vi "run.vi"(8 "error in (no error)":errorcluster, 11 "ScanHeadMH100729FPGA in":refnum<class "ScanHeadMH100729FPGA.lvclass">) -> (0 "error out":errorcluster, 3 "ScanHeadMH100729FPGA out":refnum<class "ScanHeadMH100729FPGA.lvclass">)   [LabVIEW 2010, in "ScanHeadMH100729FPGA.lvclass"]
uses:
  ScanHeadMH100729FPGA.lvclass
  intensity_adjustment_enum.ctl
  translation_mode_enum.ctl
  main/labview_source/controls/undock_button.ctl
  internal_trigger_enum.ctl
  ScanHeadMH100729FPGA.lvclass/ScanHeadMH100729FPGA.ctl
  GenericScanHead/GenericScanHead/GenericScanHead.lvclass
  Trajectory/GenericTrajectory/GenericTrajectory/GenericTrajectory.lvclass
  Trajectory/TrajectoryMG100122GenericFPGA/TrajectoryMG100122GenericFPGA/TrajectoryMG100122GenericFPGA.lvclass
  Objective/GenericObjective/GenericObjective/GenericObjective.lvclass
  <vilib>/Utility/inputDevices.llb/closeMouse.vi
  <vilib>/Utility/inputDevices.llb/closeKeyboard.vi
  common/classes/ErrorController/ErrorController/class_data.vi
  <vilib>/Utility/inputDevices.llb/mouseAcquire.vi
  <vilib>/Utility/inputDevices.llb/keyboardAcquire.vi
  common/classes/ErrorController/ErrorController/ErrorController.lvclass
panel:
  in  "button:undock":T1
  in  "Tab Control":enum32{"user", "debug", "about"}(tab)
  in  "modifyButton":bool
  in  "zoom":dbl(slide)=1.0 min=1.0 max=20.0 step=0.1 scale=1.0..20.0
  in  "offset tabs":enum32{"fine", "coarse"}(tab)
  in  "x offset":dbl[unit](slide) scale format="%#_3g"
  in  "z offset":dbl[unit](slide)
  in  "y offset":dbl[unit](slide) scale format="%#_3g"
  in  "zero offset":bool
  in  "zero angles":bool
  in  "laser intensity (%)":dbl(slide)=14.5 caption="intensity (%)" min=0.001 max=100.0 step=0.1 scale=0.0..100.0
  in  "intensity adjustment mode":T2=enum."look-up" caption="laser intensity\nadjustment"
  in  "scattering length":dbl[unit]=0.00019999999999999998 min=1e-10
  in  "z angle":dbl[unit](slide) min=0.0 max=6.283185307179586 step=0.01745329238474369
  in  "x angle":dbl[unit](slide) caption="X amplitude" min=0.0 max=3.141592653589793 step=0.01745329238474369
  in  "translation mode":T3
  in  "stop":bool
  out "evt lp error":errorcluster
  out "last trigger":T4
  out "state machine counter":i32
  # "translation"
  # "rotation & tilting"
  # "ScanHeadMH100729FPGA"
  # "Author: Marcel van 't Hoff, University of Zurich"
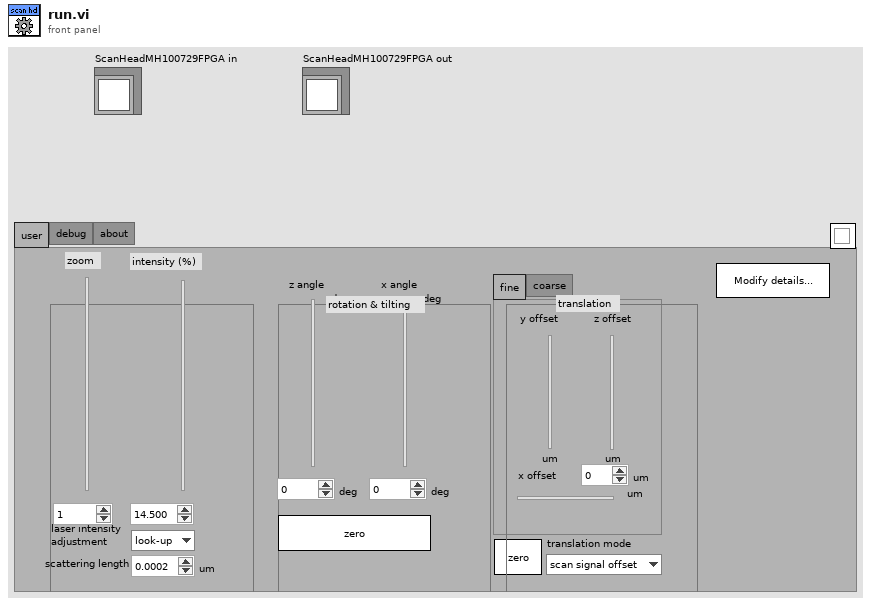
[diagram p1: front panel]
types:
  T1 = typedef "undock_button.ctl" = bool
  T2 = typedef "ScanHeadMH100729FPGA.lvclass/intensity_adjustment_enum.ctl" = enum16{"manual", "look-up", "exponential"}
  T3 = typedef "ScanHeadMH100729FPGA.lvclass/translation_mode_enum.ctl" = enum16{"scan signal offset", "stage"}
  T4 = typedef "ScanHeadMH100729FPGA.lvclass/internal_trigger_enum.ctl" = enum16{"NULL", "initialise", "terminate", "start scanning", "stop scanning", "update", "fetch trajectory", "update bounding box"}
  T5 = cluster{"Horizontal":i32, "Vertical":i32, "Scrolling":i32}
  T6 = enum16{"0", "1", "2", "3", "4", "5", "6", "7", "8", "9", "A", "B", "C", "D", "E", "F", "G", "H", "I", "J", "K", "L", "M", "N", "O", "P", "Q", "R", "S", "T", "U", "V", "W", "X", "Y", "Z", "F1", "F2", "F3", "F4", "F5", "F6", "F7", "F8", "F9", "F10", "F11", "F12", "F13", "F14", "F15", "ADD", "BACK", "BACKSLASH", "CAPITAL", "COMMA", "DECIMAL", "DELETE", "DIVIDE", "DOWN", "END", "EQUALS", "ESCAPE", "GRAVE (`)", "HOME", "INSERT", "LBRACKET", "LCONTROL", "LEFT", "L ALT", "LSHIFT", "LWIN", "MINUS", "MULTIPLY", "NEXT", "NUMLOCK", "NUMPAD_0", "NUMPAD_1", "NUMPAD_2", "NUMPAD_3", "NUMPAD_4", "NUMPAD_5", "NUMPAD_6", "NUMPAD_7", "NUMPAD_8", "NUMPAD_9", "PAUSE", "PERIOD", "PRIOR (PG UP)", "RBRACKET", "RCONTROL", "RETURN", "RIGHT", "R ALT", "RSHIFT", "RWIN", "SCROLL", "SEMICOLON", "SLASH", "SPACE", "SUBTRACT", "TAB", "UP", "ENTER (num pad)", "' (quote)"}[]
  T7 = typedef "top-level_component_type_enum.ctl" = enum16{"undefined", "ImagingMode", "ScanHead", "DAQ", "ImageAssembler", "Display", "DataCollection", "Analyser", "Stimulator", "ExperimentController", "Instrument", "Stage"}
  T8 = typedef "main_trigger_enum.ctl" = enum16{"NULL", "initialise", "terminate", "start", "stop", "change objective", "change experimentController", "change imagingMode", "save notebook", "started saving", "finished saving", "expCtr ready", "expCtr missing", "imgMd ready", "imgMd missing", "scanHd ready", "scanHd missing", "DAQ ready", "DAQ missing", "imgAsm ready", "imgAsm missing", "dataColl ready", "dataColl missing", "display ready", "display missing", "analysr ready", "analysr missing", "instrmnt ready", "instrmnt missing", "stimltr ready", "stimltr missing", "stage ready", "stage missing"}
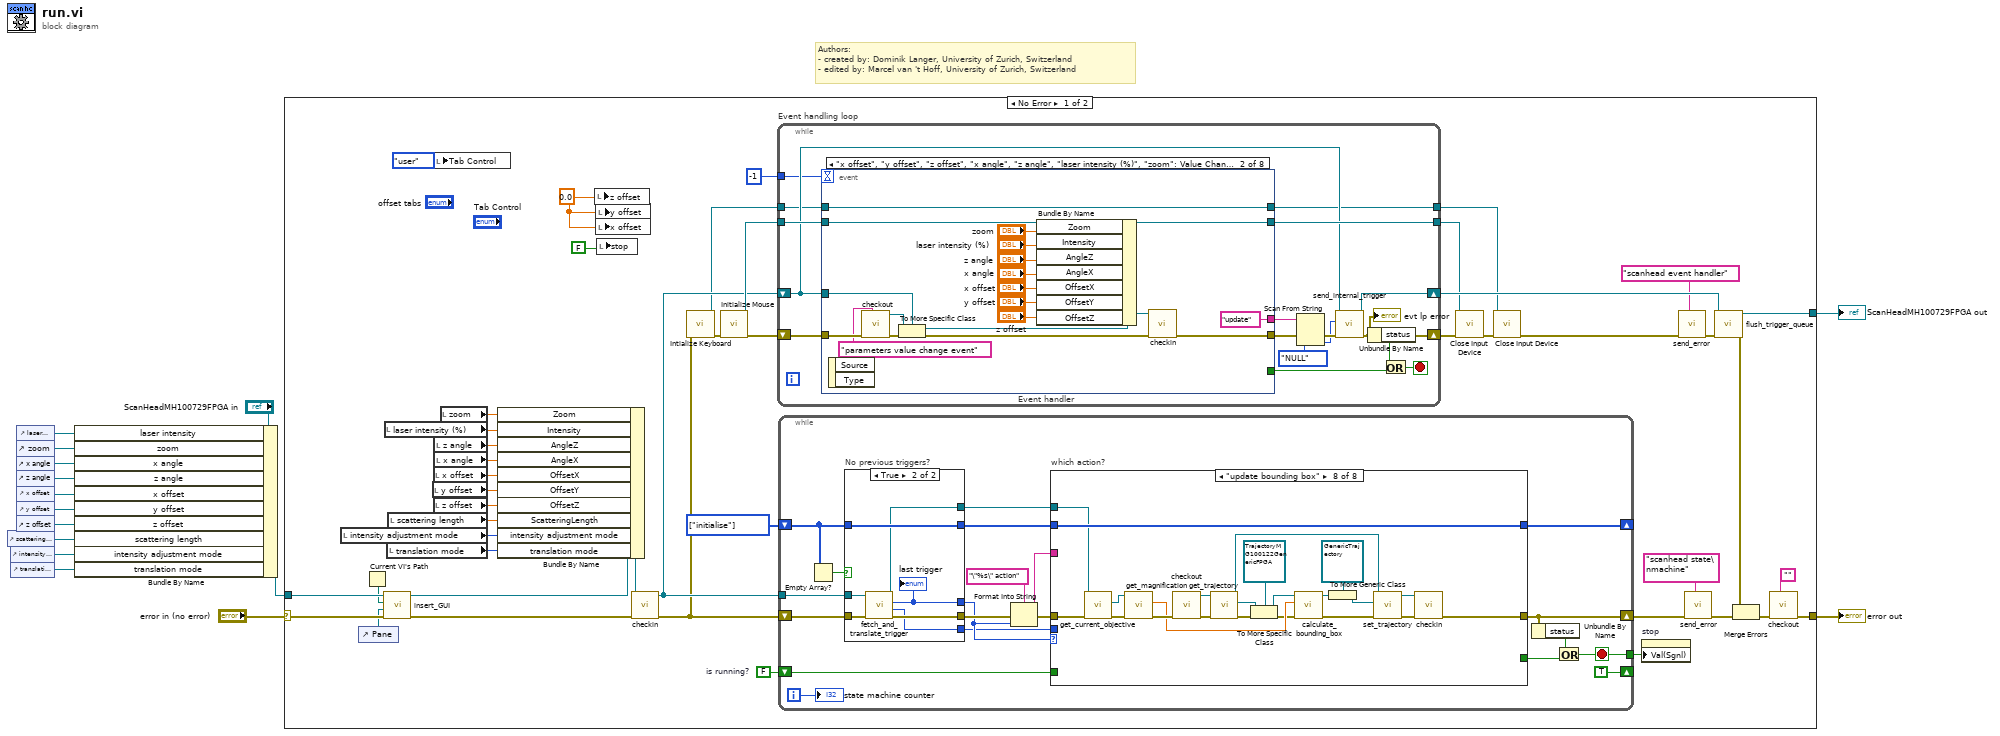
[diagram p0: block diagram]
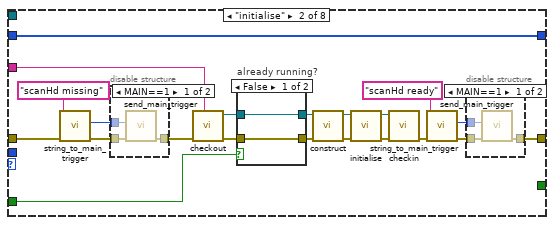
[diagram p3: hidden frame]
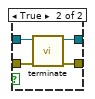
[diagram p5: hidden frame]
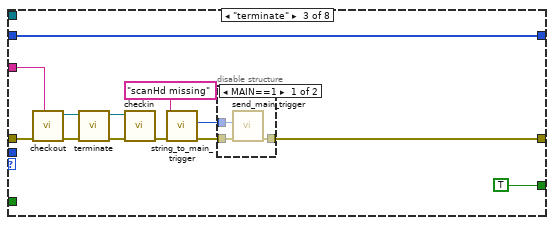
[diagram p7: hidden frame]
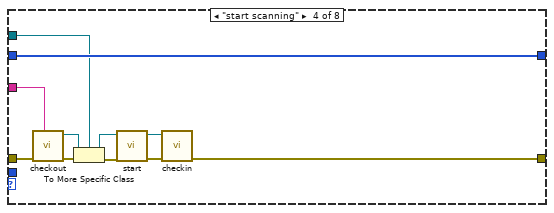
[diagram p9: hidden frame]
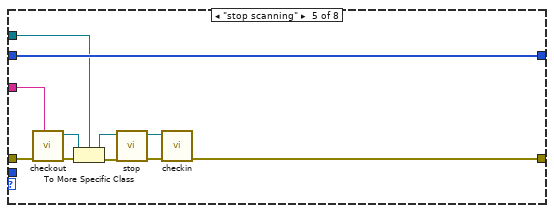
[diagram p10: hidden frame]
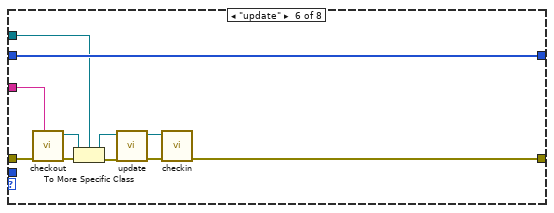
[diagram p11: hidden frame]
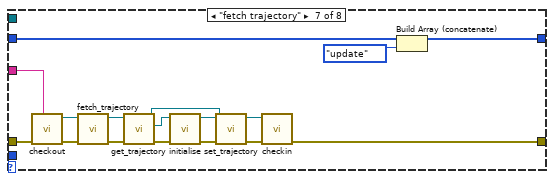
[diagram p12: hidden frame]
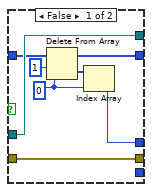
[diagram p13: hidden frame]
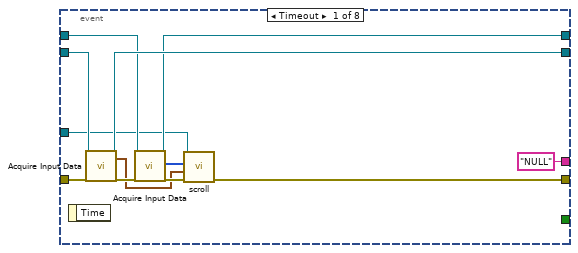
[diagram p14: hidden frame]
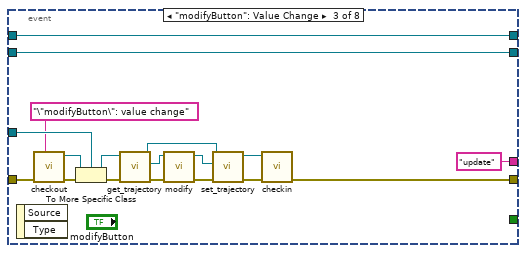
[diagram p15: hidden frame]
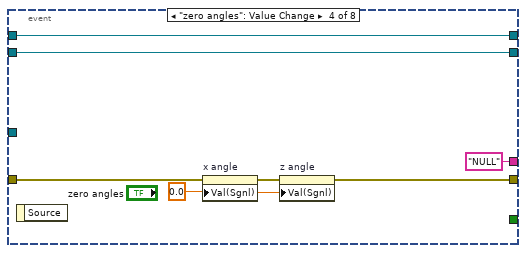
[diagram p16: hidden frame]
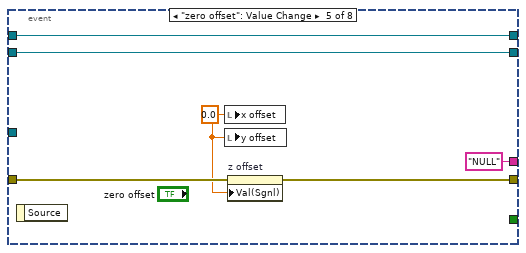
[diagram p17: hidden frame]
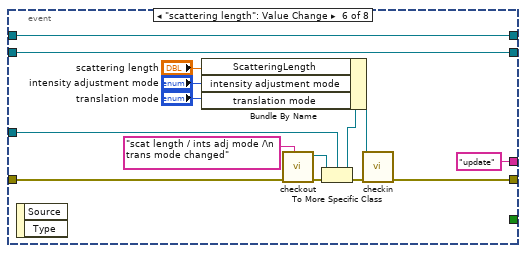
[diagram p18: hidden frame]
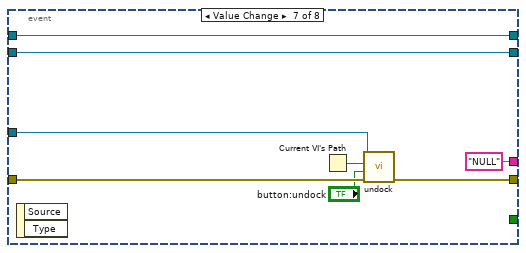
[diagram p19: hidden frame]
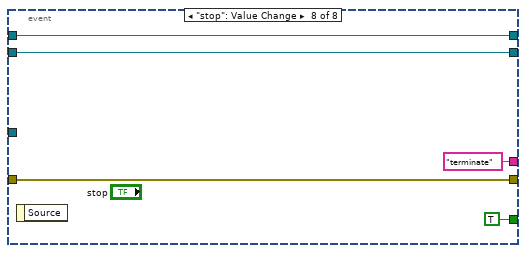
[diagram p20: hidden frame]
diagram:
  # "Authors: \n- created by: Dominik Langer, University of Zurich, Switzerland\n- edited by: Marcel van 't Hoff, University of Zurich, Switzerland"
  n1 = control-ref of="scattering length"() -> (w10:refnum<vi>)
  n2 = control-ref of="intensity adjustment mode"() -> (w9:refnum<vi>)
  n3 = control-ref of="translation mode"() -> (w3:refnum<vi>)
  n4 = control-ref of="laser intensity (%)"() -> (w8:refnum<vi>)
  n5 = control-ref of="zoom"() -> (w13:refnum<vi>)
  n6 = control-ref of="x angle"() -> (w11:refnum<vi>)
  n7 = control-ref of="z angle"() -> (w12:refnum<vi>)
  n8 = control-ref of="x offset"() -> (w5:refnum<vi>)
  n9 = control-ref of="y offset"() -> (w6:refnum<vi>)
  n10 = control-ref of="z offset"() -> (w7:refnum<vi>)
  n11 = Bundle By Name(cluster="ScanHeadMH100729FPGA in", "laser intensity"=w8, "zoom"=w13, "x angle"=w11, "z angle"=w12, "x offset"=w5, "y offset"=w6, "z offset"=w7, "scattering length"=w10, "intensity adjustment mode"=w9, "translation mode"=w3) -> (w14:refnum<class "ScanHeadMH100729FPGA.lvclass">)
  n12 = case shown="No Error" "error in (no error)" {
    selector: "error in (no error)" -> [w44 w331]
    tunnel: [w60 w331] -> w4
    tunnel: [w37 w330] -> w1
    tunnel: w14 -> [w43 w330]
    frame No Error {
      w29 = FALSE  # is running?
      w30 = T4[] [enum."initialise"] items=["NULL", "initialise", "terminate", "start scanning", "stop scanning", "update", "fetch trajectory", "update bounding box"]
      w56 = dbl[unit] 0.0 ("z offset")
      n13 = local read "intensity adjustment mode"() -> (w51:T2)
      n14 = control-ref of="Pane"() -> (w39:refnum<vi>)
      n15 = Current VI's Path() -> (path=w42:path)
      n16 = call-dynamic "insert_GUI.vi"("error in (no error)"=w44, "Pane"=w39, "VI path"=w42, "GenericComponent in"=w43) -> ("error out"=w16:errorcluster, "GenericComponent out"=w35:refnum<class "ScanHeadMH100729FPGA.lvclass">)  [unwired: 6 in]
      n17 = local read "laser intensity (%)"() -> (w53:dbl)
      n18 = local read "translation mode"() -> (w41:T3)
      n19 = local read "scattering length"() -> (w50:dbl[unit])
      n20 = local read "y offset"() -> (w46:dbl[unit])
      n21 = local read "x offset"() -> (w47:dbl[unit])
      n22 = local read "z offset"() -> (w45:dbl[unit])
      n23 = local write "Tab Control"(enum32{"user", "debug", "about"}."user" ("Tab Control")) -> ()
      n24 = local read "z angle"() -> (w49:dbl[unit])
      n25 = local read "x angle"() -> (w48:dbl[unit])
      n26 = local read "zoom"() -> (w54:dbl)
      n27 = Bundle By Name(cluster=w35, "Zoom"=w54, "Intensity"=w53, "AngleZ"=w49, "AngleX"=w48, "OffsetX"=w47, "OffsetY"=w46, "OffsetZ"=w45, "ScatteringLength"=w50, "intensity adjustment mode"=w51, "translation mode"=w41) -> (w52:refnum<class "ScanHeadMH100729FPGA.lvclass">)
      n28 = local write "z offset"(w56) -> ()
      n29 = local write "y offset"(w56) -> ()
      n30 = local write "x offset"(w56) -> ()
      n31 = local write "stop"(FALSE) -> ()
      n32 = call-dynamic "checkin.vi"("error in (no error)"=w16, "GenericScanHead in"=w52) -> ("error out"=w28:errorcluster, "GenericScanHead out"=w32:refnum<class "ScanHeadMH100729FPGA.lvclass">)  [unwired: 8 in]
      n33 = call <vilib>:"Intialize Keyboard.vi"("error in (no error)"=w28) -> ("error out"=w27:errorcluster, "device ID"=w26:refnum<k1>)  [unwired: 9 in]
      n34 = call <vilib>:"Initialize Mouse.vi"("error in (no error)"=w27) -> ("error out"=w55:errorcluster, "device ID"=w59:refnum<k1>)  [unwired: 9 in]
      n35 = while "Event handling loop" {
        shift-right: [w234] -> w21
        shift-left: w55 -> [w239]
        tunnel: w59 -> [w238]
        tunnel: [w237] -> w24
        shift-right: [w236] -> w36
        shift-left: w32 -> [w235]
        tunnel: w26 -> [w230]
        tunnel: [w229] -> w23
        tunnel: -1 -> [w228]
        stop <- w231 stop-if-true
        n36 = event "Event handler" shown="[1] \"x offset\", \"y offset\", \"z offset\", \"x angle\", \"z angle\", \"laser intensity (%)\", \"zoom\": Value Change" {
          selector: _ -> [_ _ _ _ _ _ _ _]
          dyn-events: _ -> [_ _ _ _ _ _ _ _]
          timeout: w228 -> [_ _ _ _ _ _ _ _]
          tunnel: w239 -> [w249 w268 w287 w295 w301 w306 w322 w329]
          tunnel: [w243 w258 w280 w293 w300 w305 w321 w329] -> w225
          tunnel: [_ _ _ _ _ _ _ TRUE] -> w232
          tunnel: w235 -> [w244 w267 w284 _ _ w312 w323 _]
          tunnel: w238 -> [w251 w270 w288 w291 w298 w316 w324 w327]
          tunnel: [w250 w270 w288 w291 w298 w316 w324 w327] -> w237
          tunnel: w230 -> [w247 w253 w272 w290 w297 w303 w318 w326]
          tunnel: [w246 w253 w272 w290 w297 w303 w318 w326] -> w229
          tunnel: ["NULL" "update" "update" "NULL" "NULL" "update" "NULL" "terminate"] -> w223
          event Timeout {
            n37 = event-data() -> ()  [unwired: 2 out]
            n38 = call-poly <vilib>:"Acquire Input Data.vi"("device ID"=w251, "error in (no error)"=w249) -> ("device ID"=w250:refnum<k1>, "axis info"=w241:T5, "error out"=w248:errorcluster)  [unwired: 14 in, 1 out]
            n39 = call-poly <vilib>:"Acquire Input Data.vi"("device ID"=w247, "error in (no error)"=w248) -> ("device ID"=w246:refnum<k1>, "keys pressed"=w242:T6, "error out"=w245:errorcluster)  [unwired: 15 in]
            n40 = call-dynamic "scroll.vi"("error in (no error)"=w245, "axis info"=w241, "keys pressed"=w242, "ScanHeadMH100729FPGA in"=w244) -> ("error out"=w243:errorcluster)  [unwired: 6 in, 1 out]
          }
          event "x offset", "y offset", "z offset", "x angle", "z angle", "laser intensity (%)", "zoom": Value Change {
            n41 = event-data() -> ()  [unwired: 3 out]
            n42 = call "checkout.vi"("locked by?"="parameters value change event", "error in (no error)"=w268) -> ("error out"=w269:errorcluster, "GenericScanHead out"=w266:refnum<class "GenericScanHead.lvclass">)  [unwired: 8 in]
            n43 = To More Specific Class(target class=w267, reference=w266, error in=w269) -> (specific class reference=w264:refnum<class "ScanHeadMH100729FPGA.lvclass">, error out=w259:errorcluster)
            n44 = Bundle By Name(cluster=w264, "Zoom"="zoom", "Intensity"="laser intensity (%)", "AngleZ"="z angle", "AngleX"="x angle", "OffsetX"="x offset", "OffsetY"="y offset", "OffsetZ"="z offset") -> (w257:refnum<class "ScanHeadMH100729FPGA.lvclass">)
            n45 = call-dynamic "checkin.vi"("error in (no error)"=w259, "GenericScanHead in"=w257) -> ("error out"=w258:errorcluster)  [unwired: 8 in, 1 out]
          }
          event "modifyButton": Value Change {
            n46 = event-data() -> ()  [unwired: 3 out]
            n47 = call "checkout.vi"("locked by?"="\"modifyButton\": value change", "error in (no error)"=w287) -> ("error out"=w286:errorcluster, "GenericScanHead out"=w285:refnum<class "GenericScanHead.lvclass">)  [unwired: 8 in]
            n48 = To More Specific Class(target class=w284, reference=w285, error in=w286) -> (specific class reference=w283:refnum<class "ScanHeadMH100729FPGA.lvclass">, error out=w282:errorcluster)
            n49 = call-dynamic "get_trajectory.vi"("error in (no error)"=w282, "GenericScanHead.lvclass in"=w283) -> ("error out"=w276:errorcluster, "trajectory"=w274:refnum<class "GenericTrajectory.lvclass">, "GenericScanHead.lvclass out"=w278:refnum<class "ScanHeadMH100729FPGA.lvclass">)  [unwired: 7 in]
            n50 = call-dynamic "modify.vi"("error in (no error)"=w276, "GenericTrajectory in"=w274) -> ("error out"=w275:errorcluster, "GenericTrajectory out"=w273:refnum<class "GenericTrajectory.lvclass">)  [unwired: 8 in]
            n51 = call-dynamic "set_trajectory.vi"("error in (no error)"=w275, "trajectory"=w273, "GenericScanHead.lvclass in"=w278) -> ("error out"=w281:errorcluster, "GenericScanHead.lvclass out"=w279:refnum<class "ScanHeadMH100729FPGA.lvclass">)  [unwired: 7 in]
            n52 = call-dynamic "checkin.vi"("error in (no error)"=w281, "GenericScanHead in"=w279) -> ("error out"=w280:errorcluster)  [unwired: 8 in, 1 out]
          }
          event "zero angles": Value Change {
            w292 = dbl[unit] 0.0 ("Value (Signaling)")
            n53 = event-data() -> ()  [unwired: 2 out]
            n54 = property on="x angle" class="Slide (strict)"(error in=w295, "Val(Sgnl)"=w292) -> (error out=w294:errorcluster)  [unwired: 1 in, 1 out]
            n55 = property on="z angle" class="Slide (strict)"(error in=w294, "Val(Sgnl)"=w292) -> (error out=w293:errorcluster)  [unwired: 1 in, 1 out]
          }
          event "zero offset": Value Change {
            w299 = dbl[unit] 0.0 ("x offset")
            n56 = event-data() -> ()  [unwired: 2 out]
            n57 = local write "x offset"(w299) -> ()
            n58 = local write "y offset"(w299) -> ()
            n59 = property on="z offset" class="Slide (strict)"(error in=w301, "Val(Sgnl)"=w299) -> (error out=w300:errorcluster)  [unwired: 1 in, 1 out]
          }
          event "scattering length": Value Change {
            n60 = event-data() -> ()  [unwired: 3 out]
            n61 = call "checkout.vi"("locked by?"="scat length / ints adj mode /\n trans mode changed", "error in (no error)"=w306) -> ("error out"=w309:errorcluster, "GenericScanHead out"=w311:refnum<class "GenericScanHead.lvclass">)  [unwired: 8 out]
            n62 = To More Specific Class(target class=w312, reference=w311, error in=w309) -> (specific class reference=w310:refnum<class "ScanHeadMH100729FPGA.lvclass">, error out=w308:errorcluster)
            n63 = Bundle By Name(cluster=w310, "ScatteringLength"="scattering length", "intensity adjustment mode"="intensity adjustment mode", "translation mode"="translation mode") -> (w307:refnum<class "ScanHeadMH100729FPGA.lvclass">)
            n64 = call-dynamic "checkin.vi"("error in (no error)"=w308, "GenericScanHead in"=w307) -> ("error out"=w305:errorcluster)  [unwired: 8 in, 1 out]
          }
          event Value Change {
            n65 = event-data() -> ()  [unwired: 3 out]
            n66 = Current VI's Path() -> (path=w319:path)
            n67 = call-dynamic "undock.vi"("error in (no error)"=w322, "undock?"="button:undock", "VI path"=w319, "component in"=w323) -> ("error out"=w321:errorcluster)  [unwired: 6 in, 1 out]
          }
          event "stop": Value Change {
            n68 = event-data() -> ()  [unwired: 2 out]
          }
        }
        n69 = Scan From String(input string=w223, error in=w225, default 1=internal_trigger_enum."NULL" ("trigger")) -> (error out=w226:errorcluster, output 1=w224:T4)  [unwired: 2 in, 2 out]
        n70 = call-dynamic "send_internal_trigger.vi"("error in (no error)"=w226, "trigger"=w224, "ScanHeadMH100729FPGA in"=w235) -> ("error out"=w234:errorcluster, "ScanHeadMH100729FPGA out"=w236:refnum<class "ScanHeadMH100729FPGA.lvclass">)  [unwired: 7 in]
        "evt lp error" <- w234
        n71 = Unbundle By Name(w234) -> ("status"=w233:bool)
        n72 = Or(x=w233, y=w232) -> (x .or. y?=w231:bool)
      }
      n73 = while {
        shift-right: [w66] -> w31
        shift-left: w28 -> [w81]
        shift-right: [w72] -> _
        shift-left: w30 -> [w78]
        shift-right: [TRUE ("is running?")] -> _
        shift-left: w29 -> [w69]
        tunnel: w32 -> [w80]
        tunnel: [w64] -> w18
        i -> [w62]
        stop <- w64 stop-if-true
        n74 = Empty Array?(array=w78) -> (empty?=w79:bool)
        n75 = case "No previous triggers?" shown="True" w79 {
          tunnel: w80 -> [w215 w220]
          tunnel: w81 -> [w213 w221]
          tunnel: [w215 w219] -> w73
          tunnel: [w211 w216] -> w75
          tunnel: [_ w217] -> w67
          tunnel: [w213 w218] -> w76
          tunnel: w78 -> [w214 w222]
          tunnel: [w210 w222] -> w71
          frame False {
            w208 = 0 ("index")
            n76 = Delete From Array(array=w214, length=1, index=w208) -> (deleted portion=w212:T4[], array with subset deleted=w210:T4[])
            n77 = Index Array(array=w212, index=w208) -> (element=w211:T4)
          }
          frame True {
            n78 = call-dynamic "fetch_and_translate_trigger.vi"("error in (no error)"=w221, "ScanHeadMH100729FPGA in"=w220) -> ("error out"=w218:errorcluster, "sender TLC type"=w217:T7, "internal trigger"=w216:T4, "ScanHeadMH100729FPGA out"=w219:refnum<class "ScanHeadMH100729FPGA.lvclass">)  [unwired: 6 in]
            "last trigger" <- w216
          }
        }
        n79 = Format Into String(format string="\"%s\" action", error in=w76, w75) -> (resulting string=w70:string, error out=w74:errorcluster)  [unwired: 1 in]
        n80 = case "which action?" shown="\"update bounding box\"" w75 {
          tunnel: [w82 w98 w119 w141 w152 w158 w179 w199] -> w66
          tunnel: w74 -> [w82 w85 w128 w142 w153 w164 w180 w205]
          tunnel: w73 -> [_ _ _ w138 w149 w161 _ w206]
          tunnel: [w83 w104 w131 w146 w157 w168 w170 w207] -> w72
          tunnel: w71 -> [w83 w104 w131 w146 w157 w168 w171 w207]
          tunnel: w70 -> [_ w99 w127 w140 w151 w163 w172 _]
          tunnel: w69 -> [_ w94 _ _ _ _ _ _]
          tunnel: w67 -> [_ _ _ _ _ _ _ _]
          tunnel: [_ _ TRUE _ _ _ _ _] -> w63
          frame "NULL", Default {
          }
          frame "initialise" {
            n81 = call "string_to_main_trigger.vi"("error in (no error)"=w85, "trigger string"="scanHd missing") -> ("error out"=w87:errorcluster, "main trigger"=w88:T8)  [unwired: 8 in]
            n82 = disable-structure shown="MAIN==1" {
              disable-tunnel: w87 -> [w107 w108]
              disable-tunnel: [w106 w108] -> w84
              disable-tunnel: w88 -> [w105 _]
              frame condition #0 {
                n83 = call "send_main_trigger.vi"("error in (no error)"=w107, "trigger"=w105) -> ("error out"=w106:errorcluster)  [unwired: 9 in]
              }
              frame condition #1 (active) {
              }
            }
            n84 = call "checkout.vi"("locked by?"=w99, "error in (no error)"=w84) -> ("error out"=w96:errorcluster, "GenericScanHead out"=w95:refnum<class "GenericScanHead.lvclass">)  [unwired: 8 in]
            n85 = case "already running?" shown="False" w94 {
              tunnel: [w110 w112] -> w97
              tunnel: w96 -> [w110 w111]
              tunnel: w95 -> [w109 w114]
              tunnel: [w109 w113] -> w93
              frame False {
              }
              frame True {
                n86 = call-dynamic "terminate.vi"("error in (no error)"=w111, "GenericPlugin in"=w114) -> ("error out"=w112:errorcluster, "GenericPlugin out"=w113:refnum<class "GenericScanHead.lvclass">)  [unwired: 8 out]
              }
            }
            n87 = call-dynamic "construct.vi"("error in (no error)"=w97, "GenericPlugin in"=w93) -> ("error out"=w101:errorcluster, "GenericPlugin out"=w102:refnum<class "GenericScanHead.lvclass">)  [unwired: 8 in]
            n88 = call-dynamic "initialise.vi"("error in (no error)"=w101, "GenericPlugin in"=w102) -> ("error out"=w100:errorcluster, "GenericPlugin out"=w103:refnum<class "GenericScanHead.lvclass">)  [unwired: 8 in]
            n89 = call-dynamic "checkin.vi"("error in (no error)"=w100, "GenericScanHead in"=w103) -> ("error out"=w92:errorcluster)  [unwired: 8 in, 1 out]
            n90 = call "string_to_main_trigger.vi"("error in (no error)"=w92, "trigger string"="scanHd ready") -> ("error out"=w91:errorcluster, "main trigger"=w89:T8)  [unwired: 8 in]
            n91 = disable-structure shown="MAIN==1" {
              disable-tunnel: w91 -> [w117 w118]
              disable-tunnel: [w116 w118] -> w98
              disable-tunnel: w89 -> [w115 _]
              frame condition #0 {
                n92 = call "send_main_trigger.vi"("error in (no error)"=w117, "trigger"=w115) -> ("error out"=w116:errorcluster)  [unwired: 9 in]
              }
              frame condition #1 (active) {
              }
            }
          }
          frame "terminate" {
            n93 = call "checkout.vi"("locked by?"=w127, "error in (no error)"=w128) -> ("error out"=w130:errorcluster, "GenericScanHead out"=w125:refnum<class "GenericScanHead.lvclass">)  [unwired: 8 in]
            n94 = call-dynamic "terminate.vi"("error in (no error)"=w130, "GenericPlugin in"=w125) -> ("error out"=w129:errorcluster, "GenericPlugin out"=w126:refnum<class "GenericScanHead.lvclass">)  [unwired: 8 in]
            n95 = call-dynamic "checkin.vi"("error in (no error)"=w129, "GenericScanHead in"=w126) -> ("error out"=w120:errorcluster)  [unwired: 8 in, 1 out]
            n96 = call "string_to_main_trigger.vi"("error in (no error)"=w120, "trigger string"="scanHd missing") -> ("error out"=w122:errorcluster, "main trigger"=w123:T8)  [unwired: 8 in]
            n97 = disable-structure shown="MAIN==1" {
              disable-tunnel: w122 -> [w134 w135]
              disable-tunnel: [w133 w135] -> w119
              disable-tunnel: w123 -> [w132 _]
              frame condition #0 {
                n98 = call "send_main_trigger.vi"("error in (no error)"=w134, "trigger"=w132) -> ("error out"=w133:errorcluster)  [unwired: 9 in]
              }
              frame condition #1 (active) {
              }
            }
          }
          frame "start scanning" {
            n99 = call "checkout.vi"("locked by?"=w140, "error in (no error)"=w142) -> ("error out"=w145:errorcluster, "GenericScanHead out"=w139:refnum<class "GenericScanHead.lvclass">)  [unwired: 8 in]
            n100 = To More Specific Class(target class=w138, reference=w139, error in=w145) -> (specific class reference=w137:refnum<class "ScanHeadMH100729FPGA.lvclass">, error out=w144:errorcluster)
            n101 = call-dynamic "start.vi"("error in (no error)"=w144, "ScanHeadMH100729FPGA in"=w137) -> ("error out"=w143:errorcluster, "ScanHeadMH100729FPGA out"=w136:refnum<class "ScanHeadMH100729FPGA.lvclass">)  [unwired: 8 in]
            n102 = call-dynamic "checkin.vi"("error in (no error)"=w143, "GenericScanHead in"=w136) -> ("error out"=w141:errorcluster)  [unwired: 8 in, 1 out]
          }
          frame "stop scanning" {
            n103 = call "checkout.vi"("locked by?"=w151, "error in (no error)"=w153) -> ("error out"=w156:errorcluster, "GenericScanHead out"=w150:refnum<class "GenericScanHead.lvclass">)  [unwired: 8 in]
            n104 = To More Specific Class(target class=w149, reference=w150, error in=w156) -> (specific class reference=w148:refnum<class "ScanHeadMH100729FPGA.lvclass">, error out=w155:errorcluster)
            n105 = call-dynamic "stop.vi"("error in (no error)"=w155, "ScanHeadMH100729FPGA in"=w148) -> ("error out"=w154:errorcluster, "ScanHeadMH100729FPGA out"=w147:refnum<class "ScanHeadMH100729FPGA.lvclass">)  [unwired: 8 in]
            n106 = call-dynamic "checkin.vi"("error in (no error)"=w154, "GenericScanHead in"=w147) -> ("error out"=w152:errorcluster)  [unwired: 8 in, 1 out]
          }
          frame "update" {
            n107 = call "checkout.vi"("locked by?"=w163, "error in (no error)"=w164) -> ("error out"=w167:errorcluster, "GenericScanHead out"=w162:refnum<class "GenericScanHead.lvclass">)  [unwired: 8 in]
            n108 = To More Specific Class(target class=w161, reference=w162, error in=w167) -> (specific class reference=w160:refnum<class "ScanHeadMH100729FPGA.lvclass">, error out=w166:errorcluster)
            n109 = call-dynamic "update.vi"("error in (no error)"=w166, "ScanHeadMH100729FPGA in"=w160) -> ("error out"=w165:errorcluster, "ScanHeadMH100729FPGA out"=w159:refnum<class "ScanHeadMH100729FPGA.lvclass">)  [unwired: 8 in]
            n110 = call-dynamic "checkin.vi"("error in (no error)"=w165, "GenericScanHead in"=w159) -> ("error out"=w158:errorcluster)  [unwired: 8 in, 1 out]
          }
          frame "fetch trajectory" {
            n111 = call "checkout.vi"("locked by?"=w172, "error in (no error)"=w180) -> ("error out"=w181:errorcluster, "GenericScanHead out"=w178:refnum<class "GenericScanHead.lvclass">)  [unwired: 8 in]
            n112 = call-dynamic "fetch_trajectory.vi"("error in (no error)"=w181, "GenericScanHead in"=w178) -> ("error out"=w182:errorcluster, "GenericScanHead out"=w177:refnum<class "GenericScanHead.lvclass">)  [unwired: 8 in]
            n113 = call-dynamic "get_trajectory.vi"("error in (no error)"=w182, "GenericScanHead.lvclass in"=w177) -> ("error out"=w183:errorcluster, "trajectory"=w175:refnum<class "GenericTrajectory.lvclass">, "GenericScanHead.lvclass out"=w176:refnum<class "GenericScanHead.lvclass">)  [unwired: 7 in]
            n114 = call-dynamic "initialise.vi"("error in (no error)"=w183, "GenericPlugin in"=w175) -> ("error out"=w184:errorcluster, "GenericPlugin out"=w174:refnum<class "GenericTrajectory.lvclass">)  [unwired: 8 in]
            n115 = call-dynamic "set_trajectory.vi"("error in (no error)"=w184, "trajectory"=w174, "GenericScanHead.lvclass in"=w176) -> ("error out"=w185:errorcluster, "GenericScanHead.lvclass out"=w173:refnum<class "GenericScanHead.lvclass">)  [unwired: 7 in]
            n116 = call-dynamic "checkin.vi"("error in (no error)"=w185, "GenericScanHead in"=w173) -> ("error out"=w179:errorcluster)  [unwired: 8 in, 1 out]
            n117 = Build Array (concatenate)(w171, internal_trigger_enum."update" ("last trigger")) -> (w170:T4[])
          }
          frame "update bounding box" {
            n118 = call-dynamic "get_current_objective.vi"("error in (no error)"=w205, "GenericPlugin in"=w206) -> ("error out"=w203:errorcluster, "current objective"=w204:refnum<class "GenericObjective.lvclass">)  [unwired: 7 in, 1 out]
            n119 = call-dynamic "get_magnification.vi"("error in (no error)"=w203, "GenericObjective in"=w204) -> ("error out"=w202:errorcluster, "magnification"=w198:dbl)  [unwired: 7 in, 1 out]
            n120 = call "checkout.vi"("error in (no error)"=w202) -> ("error out"=w201:errorcluster, "GenericScanHead out"=w200:refnum<class "GenericScanHead.lvclass">)  [unwired: 9 in]
            n121 = call-dynamic "get_trajectory.vi"("error in (no error)"=w201, "GenericScanHead.lvclass in"=w200) -> ("error out"=w197:errorcluster, "trajectory"=w195:refnum<class "GenericTrajectory.lvclass">, "GenericScanHead.lvclass out"=w187:refnum<class "GenericScanHead.lvclass">)  [unwired: 7 in]
            n122 = To More Specific Class(target class=refnum<class "TrajectoryMG100122GenericFPGA.lvclass"> refnum ("TrajectoryMG100122GenericFPGA.lvclass"), reference=w195, error in=w197) -> (specific class reference=w194:refnum<class "TrajectoryMG100122GenericFPGA.lvclass">, error out=w196:errorcluster)
            n123 = call-dynamic "calculate_bounding_box.vi"("error in (no error)"=w196, "magnification"=w198, "TrajectoryMG100122GenericFPGA in"=w194) -> ("error out"=w188:errorcluster, "TrajectoryMG100122GenericFPGA out"=w191:refnum<class "TrajectoryMG100122GenericFPGA.lvclass">)  [unwired: 7 in]
            n124 = To More Generic Class(target class=refnum<class "GenericTrajectory.lvclass"> refnum ("GenericTrajectory.lvclass"), reference=w191) -> (generic class reference=w189:refnum<class "GenericTrajectory.lvclass">)
            n125 = call-dynamic "set_trajectory.vi"("error in (no error)"=w188, "trajectory"=w189, "GenericScanHead.lvclass in"=w187) -> ("error out"=w193:errorcluster, "GenericScanHead.lvclass out"=w186:refnum<class "GenericScanHead.lvclass">)  [unwired: 7 in]
            n126 = call-dynamic "checkin.vi"("error in (no error)"=w193, "GenericScanHead in"=w186) -> ("error out"=w199:errorcluster)  [unwired: 8 in, 1 out]
          }
        }
        n127 = Unbundle By Name(w66) -> ("status"=w65:bool)
        n128 = Or(x=w65, y=w63) -> (x .or. y?=w64:bool)
        "state machine counter" <- w62
      }
      n129 = call-poly <vilib>:"Close Input Device.vi"("error in (no error)"=w21, "device ID"=w24) -> ("error out"=w22:errorcluster)  [unwired: 8 in]
      n130 = call-poly <vilib>:"Close Input Device.vi"("error in (no error)"=w22, "device ID"=w23) -> ("error out"=w20:errorcluster)  [unwired: 8 in]
      n131 = property on="stop" class="Bool (strict)"("Val(Sgnl)"=w18) -> ()  [unwired: 2 in, 2 out]
      n132 = call "send_error.vi"("additional message"="scanhead event handler", "error in (no error)"=w20) -> ("error out"=w25:errorcluster)  [unwired: 9 in]
      n133 = call "send_error.vi"("additional message"="scanhead state\nmachine", "error in (no error)"=w31) -> ("error out"=w17:errorcluster)  [unwired: 9 in]
      n134 = call-dynamic "flush_trigger_queue.vi"("error in (no error)"=w25, "GenericToplevelComponent in"=w36) -> ("error out"=w38:errorcluster, "GenericToplevelComponent out"=w37:refnum<class "ScanHeadMH100729FPGA.lvclass">)  [unwired: 8 in]
      n135 = Merge Errors(w38, w17) -> (w58:errorcluster)
      n136 = call "checkout.vi"("locked by?"="", "error in (no error)"=w58) -> ("error out"=w60:errorcluster)  [unwired: 9 out]
    }
    frame Error {
    }
  }
  "error out" <- w4
  "ScanHeadMH100729FPGA out" <- w1
